vi "VISA Protocol FG.vi"(7 "Action":T1, 8 "error in (no error)":errorcluster, 10 "VISA Config":T2={"VISA Resource"="GPIB0::2::INSTR", "Enable Termination Character"=TRUE, "Termination Character"=10, "Timeout"=2000, "Append Write Termination Character"=FALSE} {"Termination Character" format="%.0x"}, 11 "Device Item Ref in":T3 format="%.0x") -> (0 "error out":errorcluster, 2 "VISA Config":T2={"VISA Resource"="GPIB0::2::INSTR", "Enable Termination Character"=TRUE, "Termination Character"=10, "Timeout"=10, "Append Write Termination Character"=TRUE} {"Termination Character" format="%.0x"}, 3 "Item Ref out":T3 format="%.0x")   [LabVIEW 2019, in "Instrument Addon Shared.lvlib"]
uses:
  Instrument Addon Shared.lvlib
  <vilib>/NI VeriStand/Custom Device API/Custom Device Item Ref.ctl
  Types/VISA Settings.ctl
  Types/FG Control.ctl
  Constants.vi
  <vilib>/NI VeriStand/Custom Device API/Get Item Property (Boolean).vi
  <vilib>/NI VeriStand/Custom Device API/Get Item Property (U32).vi
  <vilib>/NI VeriStand/Custom Device API/Get Item Property (String).vi
  <vilib>/NI VeriStand/Custom Device API/Set Item Property (Boolean).vi
  <vilib>/NI VeriStand/Custom Device API/Set Item Property (U32).vi
  <vilib>/NI VeriStand/Custom Device API/Set Item Property (String).vi
  <vilib>/NI VeriStand/Custom Device API/Custom Device API.lvlib
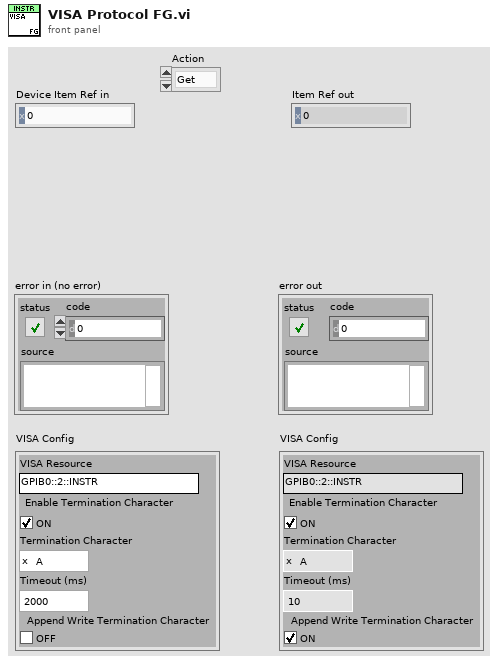
[diagram p1: front panel]
types:
  T1 = typedef "Instrument Addon Shared.lvlib/FG Control.ctl" = enum16{"Get", "Set"}
  T2 = typedef "Instrument Addon Shared.lvlib/VISA Settings.ctl" = cluster{"VISA Resource":string, "Enable Termination Character":bool, "Termination Character":u8, "Timeout":u32, "Append Write Termination Character":bool}
  T3 = typedef "Custom Device API.lvlib/Custom Device Item Ref.ctl" = u64
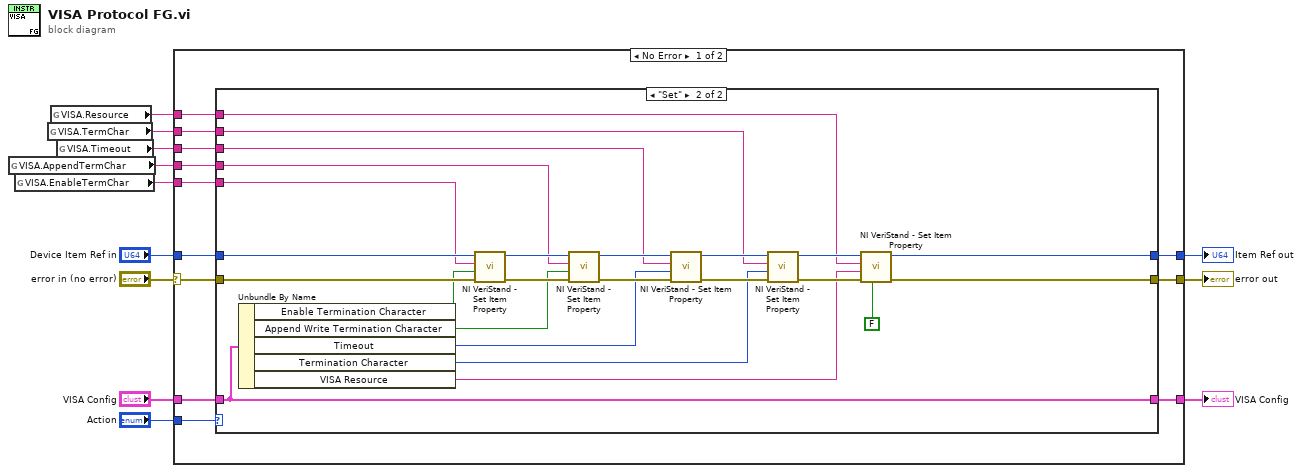
[diagram p0: block diagram]
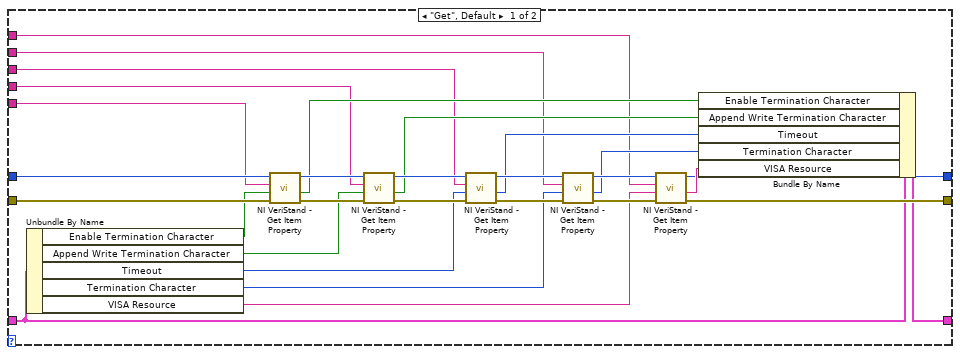
[diagram p2: hidden frame]
diagram:
  n1 = global read "Constants.vi" "VISA.AppendTermChar"() -> (w2:string)
  n2 = global read "Constants.vi" "VISA.EnableTermChar"() -> (w1:string)
  n3 = global read "Constants.vi" "VISA.TermChar"() -> (w4:string)
  n4 = global read "Constants.vi" "VISA.Resource"() -> (w12:string)
  n5 = global read "Constants.vi" "VISA.Timeout"() -> (w3:string)
  n6 = case shown="No Error" "error in (no error)" {
    selector: "error in (no error)" -> [w19 w80]
    tunnel: w12 -> [w24 _]
    tunnel: [w23 w78] -> w11
    tunnel: "Device Item Ref in" -> [w22 w78]
    tunnel: "VISA Config" -> [w21 w79]
    tunnel: [w20 w80] -> w8
    tunnel: [w18 w79] -> w6
    tunnel: "Action" -> [w17 _]
    tunnel: w4 -> [w16 _]
    tunnel: w3 -> [w15 _]
    tunnel: w2 -> [w14 _]
    tunnel: w1 -> [w13 _]
    frame No Error {
      n7 = case shown="\"Set\"" w17 {
        tunnel: w24 -> [w25 w55]
        tunnel: [w35 w67] -> w23
        tunnel: w22 -> [w52 w66]
        tunnel: w21 -> [w37 w65]
        tunnel: [w43 w68] -> w20
        tunnel: w19 -> [w53 w69]
        tunnel: [w34 w65] -> w18
        tunnel: w16 -> [w26 w59]
        tunnel: w15 -> [w27 w58]
        tunnel: w14 -> [w28 w57]
        tunnel: w13 -> [w29 w56]
        frame "Get", Default {
          n8 = Unbundle By Name(w37) -> ("Enable Termination Character"=w42:bool, "Append Write Termination Character"=w41:bool, "Timeout"=w40:u32, "Termination Character"=w39:u8, "VISA Resource"=w38:string)
          n9 = call-poly <vilib>:"NI VeriStand - Get Item Property.vi"("error in (no error)"=w53, "Default Value"=w42, "Property Name"=w29, "Item Ref in"=w52) -> ("error out"=w51:errorcluster, "Value"=w30:bool, "Item Ref out"=w47:T3)  [unwired: 4 in, 1 out]
          n10 = call-poly <vilib>:"NI VeriStand - Get Item Property.vi"("error in (no error)"=w51, "Default Value"=w41, "Property Name"=w28, "Item Ref in"=w47) -> ("error out"=w50:errorcluster, "Value"=w31:bool, "Item Ref out"=w46:T3)  [unwired: 4 in, 1 out]
          n11 = call-poly <vilib>:"NI VeriStand - Get Item Property.vi"("error in (no error)"=w50, "Default Value"=w40, "Property Name"=w27, "Item Ref in"=w46) -> ("error out"=w49:errorcluster, "Value"=w32:u32, "Item Ref out"=w45:T3)  [unwired: 4 in, 1 out]
          n12 = call-poly <vilib>:"NI VeriStand - Get Item Property.vi"("error in (no error)"=w49, "Default Value"=w39, "Property Name"=w26, "Item Ref in"=w45) -> ("error out"=w48:errorcluster, "Value"=w33:u32, "Item Ref out"=w44:T3)  [unwired: 4 in, 1 out]
          n13 = call-poly <vilib>:"NI VeriStand - Get Item Property.vi"("error in (no error)"=w48, "Default Value"=w38, "Property Name"=w25, "Item Ref in"=w44) -> ("error out"=w43:errorcluster, "Value"=w36:string, "Item Ref out"=w35:T3)  [unwired: 4 in, 1 out]
          n14 = Bundle By Name(cluster=w37, "Enable Termination Character"=w30, "Append Write Termination Character"=w31, "Timeout"=w32, "Termination Character"=w33, "VISA Resource"=w36) -> (w34:T2)
        }
        frame "Set" {
          n15 = Unbundle By Name(w65) -> ("Enable Termination Character"=w60:bool, "Append Write Termination Character"=w61:bool, "Timeout"=w62:u32, "Termination Character"=w63:u8, "VISA Resource"=w64:string)
          n16 = call-poly <vilib>:"NI VeriStand - Set Item Property.vi"("error in (no error)"=w69, "Value"=w60, "Property Name"=w56, "Item Ref in"=w66) -> ("error out"=w77:errorcluster, "Item Ref out"=w73:T3)  [unwired: 5 in, 1 out]
          n17 = call-poly <vilib>:"NI VeriStand - Set Item Property.vi"("error in (no error)"=w77, "Value"=w61, "Property Name"=w57, "Item Ref in"=w73) -> ("error out"=w76:errorcluster, "Item Ref out"=w72:T3)  [unwired: 5 in, 1 out]
          n18 = call-poly <vilib>:"NI VeriStand - Set Item Property.vi"("error in (no error)"=w76, "Value"=w62, "Property Name"=w58, "Item Ref in"=w72) -> ("error out"=w75:errorcluster, "Item Ref out"=w71:T3)  [unwired: 5 in, 1 out]
          n19 = call-poly <vilib>:"NI VeriStand - Set Item Property.vi"("error in (no error)"=w75, "Value"=w63, "Property Name"=w59, "Item Ref in"=w71) -> ("error out"=w74:errorcluster, "Item Ref out"=w70:T3)  [unwired: 5 in, 1 out]
          n20 = call-poly <vilib>:"NI VeriStand - Set Item Property.vi"("Binary String (T)"=FALSE, "error in (no error)"=w74, "Value"=w64, "Property Name"=w55, "Item Ref in"=w70) -> ("error out"=w68:errorcluster, "Item Ref out"=w67:T3)  [unwired: 4 in, 1 out]
        }
      }
    }
    frame Error {
    }
  }
  "Item Ref out" <- w11
  "error out" <- w8
  "VISA Config" <- w6
